vi "edit device on off group.vi"(9 "ItemSyms in":i32[](array[numeric]), 10 "Device Group":string, 11 "MulticolumnListbox in":refnum<vi>) -> (0 "error out":errorcluster, 3 "ItemSyms out":i32[](array[numeric]))   [LabVIEW 2020]
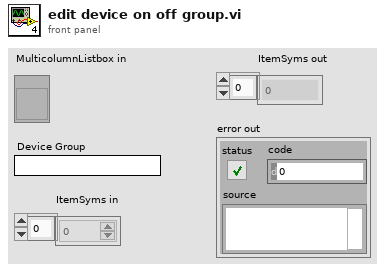
[diagram p1: front panel]
types:
  T1 = typedef "mysql_authentication.ctl" = cluster{"User":string, "Password":string, "Database":string}
  T2 = cluster{"Port":u16, "IP Address":string, "Authentication":T1}
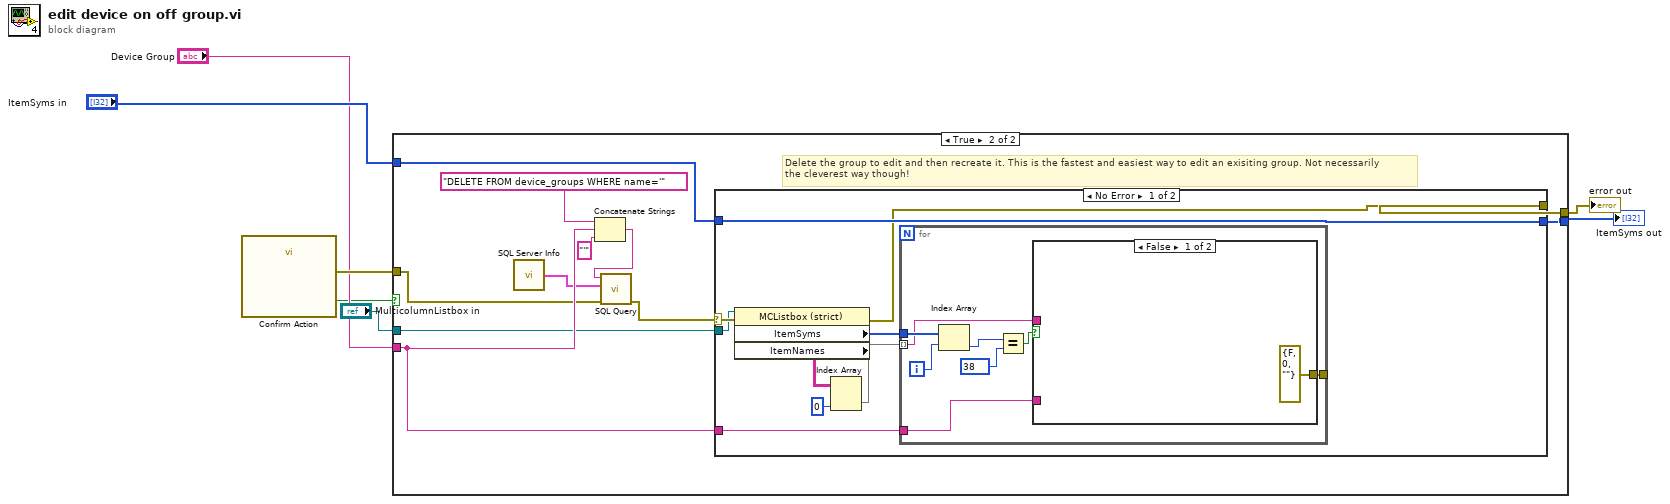
[diagram p0: block diagram]
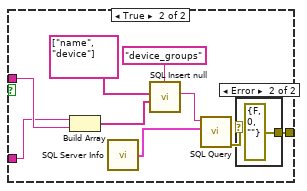
[diagram p3: hidden frame]
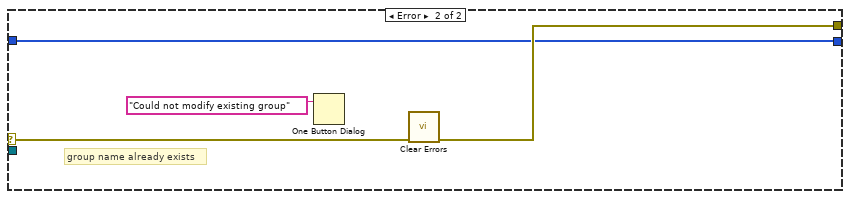
[diagram p5: hidden frame]
diagram:
  n1 = call "Confirm Action"() -> ("Edit Group"=w2:bool, "error out"=w6:errorcluster)  [unwired: 18 in]
  n2 = case shown="True" w2 {
    tunnel: "Device Group" -> [_ w19]
    tunnel: "ItemSyms in" -> [w8 w14]
    tunnel: [w8 w13] -> w5
    tunnel: w6 -> [w9 w12]
    tunnel: [w9 w11] -> w7
    tunnel: "MulticolumnListbox in" -> [_ w10]
    frame False {
    }
    frame True {
      # "Delete the group to edit and then recreate it. This is the fastest and easiest way to edit an exisiting group. Not necessarily\nthe cleverest way though!"
      n3 = call "SQL Server Info.vi"() -> ("SQL Server Info"=w17:T2)
      n4 = Concatenate Strings("DELETE FROM device_groups WHERE name='" ("Query"), w19, "'" ("string")) -> (w16:string)
      n5 = call "SQL Query.vi"("error in (no error)"=w12, "SQL Server Info"=w17, "Query"=w16) -> ("error out"=w15:errorcluster)  [unwired: 7 in, 1 out]
      n6 = case shown="No Error" w15 {
        selector: w15 -> [w23 w52]
        tunnel: w19 -> [w25 _]
        tunnel: w14 -> [w24 w50]
        tunnel: [w24 w50] -> w13
        tunnel: [w22 w51] -> w11
        tunnel: w10 -> [w21 _]
        frame No Error {
          n7 = property on="Property Node" class="MCListbox (strict)"(reference=w21, error in=w23) -> (error out=w22:errorcluster, "ItemSyms"=w27:i32[], "ItemNames"=w28:string[][])  [unwired: 1 out]
          n8 = Index Array(array=w28, index (col)=0 ("disabled index (col)")) -> (element=w26:string[])  [unwired: 1 in]
          n9 = for {
            tunnel: w26 -> [w32] mode=indexing
            tunnel: w27 -> [w36]
            tunnel: w25 -> [w31]
            tunnel: [w30] -> _
            i -> [w34]
            n10 = Index Array(array=w36, index=w34) -> (element=w35:i32)
            n11 = Equal?(x=w35, y=38) -> (x = y?=w33:bool)
            n12 = case shown="False" w33 {
              tunnel: w32 -> [_ w43]
              tunnel: w31 -> [_ w42]
              tunnel: [errorcluster {"status"=FALSE, "code"=0, "source"=""} ("error IO") w39] -> w30
              frame False {
              }
              frame True {
                n13 = Build Array(w42, w43) -> (w46:string[])
                n14 = call "SQL Server Info.vi"() -> ("SQL Server Info"=w47:T2)
                n15 = call "SQL Insert null.vi"("Values"=w46, "Column Names"=string[] ["name", "device"] ("appended array"), "Table"="device_groups") -> ("Query String"=w41:string)  [unwired: 8 in]
                n16 = call "SQL Query.vi"("SQL Server Info"=w47, "Query"=w41) -> ("error out"=w40:errorcluster)  [unwired: 8 in, 1 out]
                n17 = case shown="Error" w40 {
                  selector: w40 -> [w48 _]
                  tunnel: [w48 errorcluster {"status"=FALSE, "code"=0, "source"=""} ("error IO")] -> w39
                  frame No Error {
                  }
                  frame Error {
                  }
                }
              }
            }
          }
        }
        frame Error {
          # "group name already exists"
          n18 = One Button Dialog(message="Could not modify existing group") -> ()  [unwired: 1 in, 1 out]
          n19 = call <vilib>:"Clear Errors.vi"("error in (no error)"=w52) -> ("error out"=w51:errorcluster)  [unwired: 5 in, 1 out]
        }
      }
    }
  }
  "error out" <- w7
  "ItemSyms out" <- w5
